vi "Bool_Pulse on off.vi"(7 "Current Time":timestamp, 8 "Mode":enum16{"Delay Off", "Delay On", "Delay Both"}(ring)=enum."Delay Both", 9 "Delay Time Off":dbl=0.5 format="%.2g", 10 "Delay Time On":dbl=0.5 format="%.2g", 11 "Input":bool) -> (3 "Output Out":bool, 5 "Time Left (S) Out":dbl)   [LabVIEW 2020]
panel:
  in  "stop":bool=TRUE
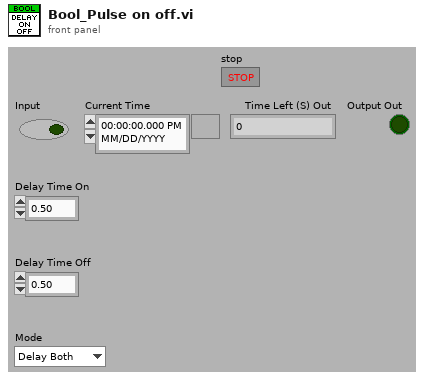
[diagram p1: front panel]
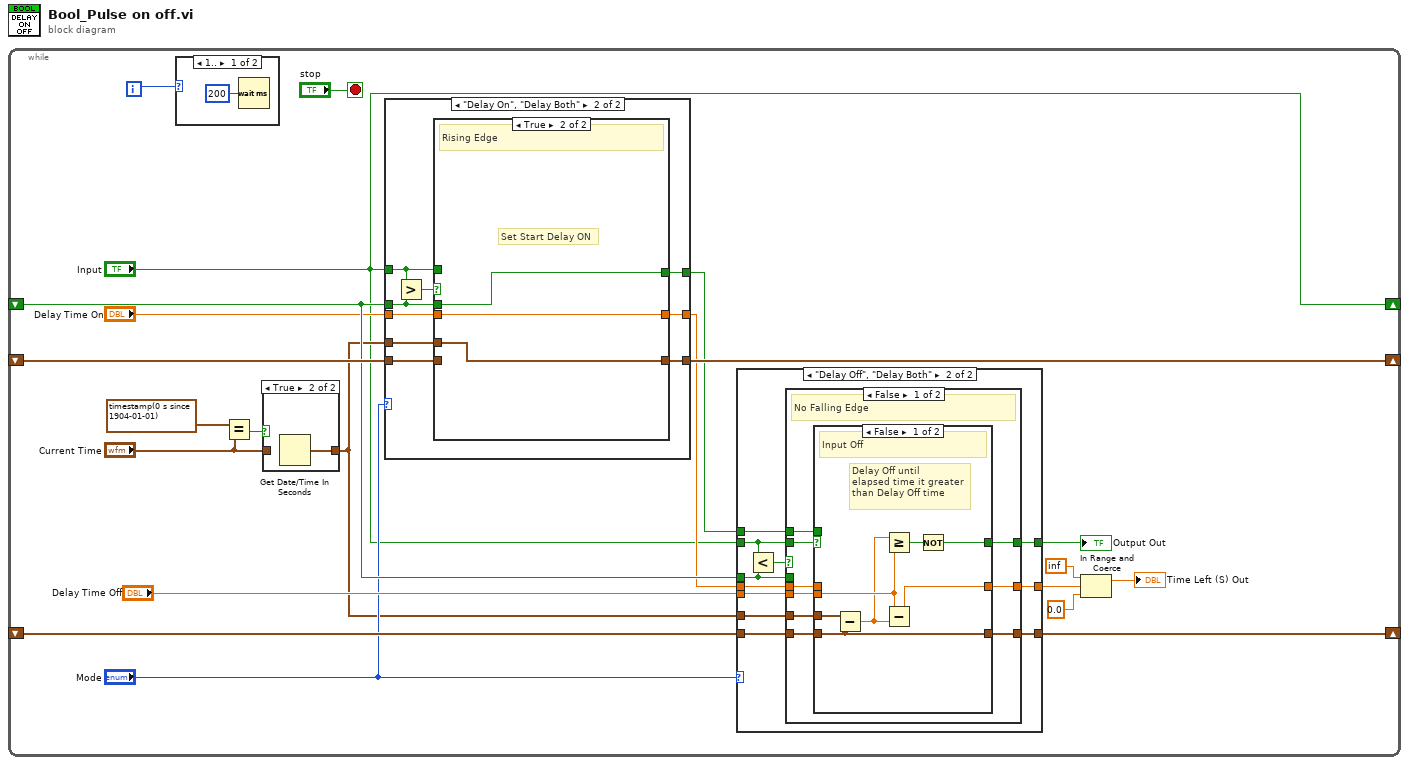
[diagram p0: block diagram]
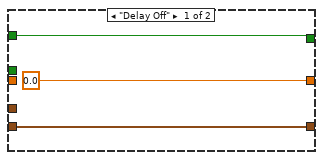
[diagram p6: hidden frame]
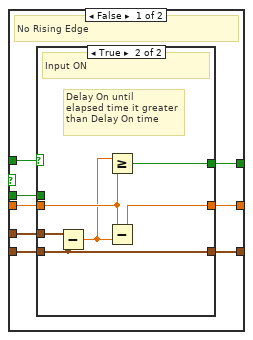
[diagram p7: hidden frame]
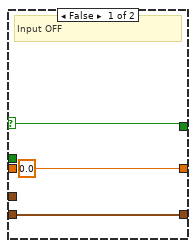
[diagram p8: hidden frame]
diagram:
  n1 = while {
    shift-right: [w20] -> _
    shift-left: _ -> [w19]
    shift-right: ["Input"] -> _
    shift-left: _ -> [w18]
    shift-right: [w16] -> _
    shift-left: _ -> [w15]
    i -> [w21]
    stop <- "stop" stop-if-true
    n2 = case shown="1.." w21 {
      frame 1.. {
        n3 = Wait (ms)(milliseconds to wait=u32 200) -> ()  [unwired: 1 out]
      }
      frame ..0 {
      }
    }
    n4 = Equal?(x=timestamp(0 s since 1904-01-01) ("Current Time"), y="Current Time") -> (x = y?=w9:bool)
    n5 = case shown="True" w9 {
      tunnel: [w23 w24] -> w7
      tunnel: "Current Time" -> [w23 _]
      frame False {
      }
      frame True {
        n6 = Get Date/Time In Seconds() -> (seconds since 1Jan1904=w24:timestamp)
      }
    }
    n7 = case shown="\"Delay On\", \"Delay Both\"" "Mode" {
      tunnel: "Input" -> [w61 w64]
      tunnel: w18 -> [_ w71]
      tunnel: "Delay Time On" -> [_ w65]
      tunnel: w7 -> [_ w69]
      tunnel: [w62 w70] -> w20
      tunnel: w19 -> [w62 w68]
      tunnel: [w61 w67] -> w1
      tunnel: [0.0 w66] -> w14
      frame "Delay Off" {
      }
      frame "Delay On", "Delay Both" {
        n8 = Greater?(x=w64, y=w71) -> (0:w72:bool)
        n9 = case shown="True" w72 {
          tunnel: w71 -> [w73 w91]
          tunnel: [w74 w92] -> w70
          tunnel: w69 -> [w80 w92]
          tunnel: w68 -> [w76 _]
          tunnel: [w79 w91] -> w67
          tunnel: [w77 w90] -> w66
          tunnel: w65 -> [w78 w90]
          tunnel: w64 -> [w75 _]
          frame False {
            # "No Rising Edge"
            n10 = case shown="True" w75 {
              selector: w75 -> [w81 _]
              tunnel: w80 -> [_ w89]
              tunnel: [w81 w88] -> w79
              tunnel: w78 -> [_ w87]
              tunnel: [0.0 w85] -> w77
              tunnel: w76 -> [w82 w84]
              tunnel: [w82 w84] -> w74
              tunnel: w73 -> [_ _]
              frame False {
                # "Input OFF"
              }
              frame True {
                # "Delay On until\nelapsed time it greater\nthan Delay On time"
                # "Input ON"
                n11 = Subtract(x=w89, y=w84) -> (x-y=w86:dbl)
                n12 = Greater Or Equal?(x=w86, y=w87) -> (x >= y?=w88:bool)
                n13 = Subtract(x=w87, y=w86) -> (x-y=w85:dbl)
              }
            }
          }
          frame True {
            # "Set Start Delay ON"
            # "Rising Edge"
          }
        }
      }
    }
    n14 = case shown="\"Delay Off\", \"Delay Both\"" "Mode" {
      tunnel: "Input" -> [_ w30]
      tunnel: w18 -> [_ w37]
      tunnel: "Delay Time Off" -> [_ w31]
      tunnel: w7 -> [_ w35]
      tunnel: [w27 w36] -> w16
      tunnel: w15 -> [w27 w34]
      tunnel: [w25 w33] -> w17
      tunnel: [w26 w32] -> w6
      tunnel: w14 -> [w26 w29]
      tunnel: w1 -> [w25 w28]
      frame "Delay On" {
      }
      frame "Delay Off", "Delay Both" {
        n15 = Less?(x=w30, y=w37) -> (x < y?=w38:bool)
        n16 = case shown="False" w38 {
          tunnel: w37 -> [_ w58]
          tunnel: [w41 w60] -> w36
          tunnel: w35 -> [w47 w60]
          tunnel: w34 -> [w43 _]
          tunnel: [w46 w58] -> w33
          tunnel: [w44 w59] -> w32
          tunnel: w31 -> [w45 w59]
          tunnel: w30 -> [w42 _]
          tunnel: w29 -> [w40 _]
          tunnel: w28 -> [w39 _]
          frame False {
            # "No Falling Edge"
            n17 = case shown="False" w42 {
              tunnel: w47 -> [w54 _]
              tunnel: [w48 w55] -> w46
              tunnel: w45 -> [w52 _]
              tunnel: [w50 w56] -> w44
              tunnel: w43 -> [w49 w57]
              tunnel: [w49 w57] -> w41
              tunnel: w40 -> [_ w56]
              tunnel: w39 -> [_ w55]
              frame False {
                # "Delay Off until\nelapsed time it greater\nthan Delay Off time"
                # "Input Off"
                n18 = Subtract(x=w54, y=w49) -> (x-y=w51:dbl)
                n19 = Greater Or Equal?(x=w51, y=w52) -> (x >= y?=w53:bool)
                n20 = Subtract(x=w52, y=w51) -> (x-y=w50:dbl)
                n21 = Not(x=w53) -> (.not. x?=w48:bool)
              }
              frame True {
                # "Input ON"
              }
            }
          }
          frame True {
            # "Set Start Delay Off"
            # "Falling Edge"
          }
        }
      }
    }
    "Output Out" <- w17
    n22 = In Range and Coerce(upper limit=inf, x=w6, lower limit=0.0) -> (coerced(x)=→"Time Left (S) Out":dbl)  [unwired: 1 out]
  }
